vi "Disconnect.vi"(8 "error in":errorcluster, 11 "2727 in":refnum<class "2727.lvclass">) -> (0 "error out":errorcluster, 3 "2727 out":refnum<class "2727.lvclass">)   [LabVIEW 2019, in "2727.lvlib" / "2727.lvclass"]
uses:
  Library/2727.lvclass
  Library/2727.lvclass/2727.ctl
  <instrlib>/ni272xReferenceVIs/ni272xReferenceVIs.llb/ni272x Reference.ctl
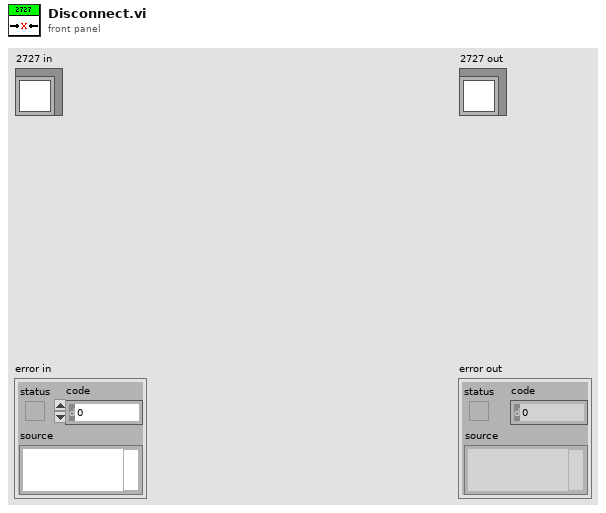
[diagram p1: front panel]
types:
  T1 = typedef "ni272x Reference.ctl" = refnum<k20>
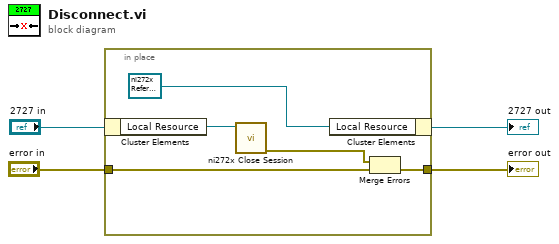
[diagram p0: block diagram]
diagram:
  n1 = in-place {
    in-place-border: "error in" -> [w6]
    in-place-border: [w5] -> w1
    n2 = in-place-cluster #1("2727 in") -> ("Local Resource"=w9:T1)
    n3 = call <instrlib>:"ni272x Close Session.vi"("instrument handle"=w9) -> ("error out"=w7:errorcluster)  [unwired: 2 in, 8 out]
    n4 = in-place-cluster #1("Local Resource"=T1 refnum) -> (→"2727 out":refnum<class "2727.lvclass">)
    n5 = Merge Errors(w7, w6) -> (w5:errorcluster)
  }
  "error out" <- w1
